vi "Get Strings from Ref.vi"(8 "error in (no error)":errorcluster, 9 "Label Prefix":string, 10 "GObj Refnum in":refnum<vi>, 11 "BoolControl in":refnum<class "BoolControl.lvclass">) -> (0 "error out":errorcluster, 1 "Valid?":bool, 2 "GObj Refnum out":refnum<vi>, 3 "BoolControl out":refnum<class "BoolControl.lvclass">, 4 "GObj Name":string)   [LabVIEW 2013, in "SET Project Data.lvlib" / "BoolControl.lvclass"]
uses:
  BoolControl.lvclass
  Control/Control.lvclass
  SET Project Data.lvlib
  GObject/GObject.lvclass
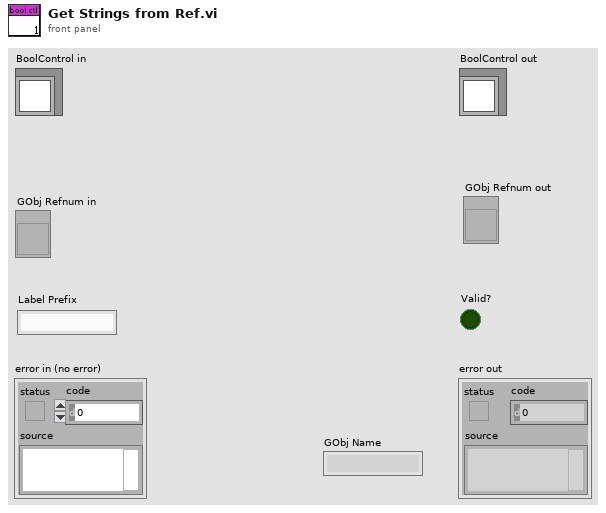
[diagram p1: front panel]
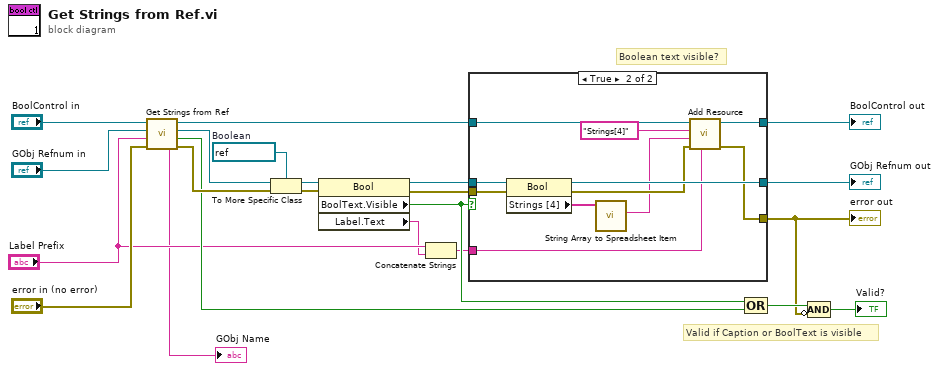
[diagram p0: block diagram]
diagram:
  w17 = refnum<vi> refnum  # Boolean
  # "Valid if Caption or BoolText is visible"
  # "Boolean text visible?"
  n1 = call-parent "Get Strings from Ref.vi"("error in (no error)"="error in (no error)", "Label Prefix"="Label Prefix", "GObj Refnum in"="GObj Refnum in", "Control in"="BoolControl in") -> ("error out"=w18:errorcluster, "Valid?"=w8:bool, "GObj Refnum out"=w19:refnum<vi>, "Control out"=w16:refnum<class "BoolControl.lvclass">, "GObj Name"=→"GObj Name":string)  [unwired: 3 in]
  n2 = To More Specific Class(target class=w17, reference=w19, error in=w18) -> (specific class reference=w13:refnum<vi>, error out=w12:errorcluster)
  n3 = property class="Bool"(reference=w13, error in=w12) -> (reference out=w11:refnum<vi>, error out=w10:errorcluster, "BoolText.Visible"=w9:bool, "Label.Text"=w3:string)
  n4 = Concatenate Strings("Label Prefix", w3) -> (w2:string)
  n5 = case shown="True" w9 {
    tunnel: w11 -> [w25 w36]
    tunnel: w16 -> [w24 w32]
    tunnel: [w24 w31] -> w15
    tunnel: [w23 w29] -> w6
    tunnel: [w25 w35] -> w14
    tunnel: w10 -> [w23 w34]
    tunnel: w2 -> [_ w30]
    frame False {
    }
    frame True {
      n6 = property class="Bool"(reference=w36, error in=w34) -> (reference out=w35:refnum<vi>, error out=w28:errorcluster, "Strings [4]"=w33:string[])
      n7 = call "String Array to Spreadsheet Item.vi"("Strings [] (ASCII)"=w33) -> ("Spreadsheet Item (ASCII)"=w27:string)  [unwired: 10 in]
      n8 = call "Add Resource.vi"("TagPrefix"=w30, "error in (no error)"=w28, "ItemText"=w27, "ItemName"="Strings[4]", "GObject in"=w32) -> ("error out"=w29:errorcluster, "GObject out"=w31:refnum<class "BoolControl.lvclass">)  [unwired: 5 in]
    }
  }
  "error out" <- w6
  "BoolControl out" <- w15
  "GObj Refnum out" <- w14
  n9 = Compound Arithmetic op=OR(w9, w8) -> (w7:bool)
  n10 = Compound Arithmetic op=AND(w7, invert w6) -> (→"Valid?":bool)
